vi "Weather_station_main.vi"() -> ()   [LabVIEW 2018]
doc: "通过datasocket技术接收weatherdata发送的数据，之后将数据进行数据显示、数据存储。"
uses:
  variable/weatherdata.vi
  variable/stop.vi
  controls/duoyun.ctl
  controls/dayu.ctl
  controls/sunshine.ctl
panel:
  in  "Array":i8[](array[numeric])
  in  "选项卡控件":enum32{"实时天气显示", "系统结构图"}(tab)
  in  "record":bool caption="停止"
  out "时间":string="21:04"
  in  "地区选择":T1(ring)=enum."金山区"
  out "风速(米/秒)":dbl(knob)=1.2703881999030089 scale=0.0..60.0
  out "风向(度)":dbl(knob)=188.40091984285937 scale=0.0..350.0
  out "气压":dbl(slide)=1004.1359589167787 scale=800.0..1100.0
  out "湿度":dbl(slide)=16.088642176316135 scale=0.0..100.0
  out "温度":dbl(slide)=30.587121929296547 caption="温度(摄氏)" scale=15.0..40.0
  out "雨量(毫米)":dbl(slide)=4.3994523493909 scale=0.0..20.0
  in  "stop":bool caption="停止"
  in  "气象数据更新":bool
  out "日期":string="2007-9-9"
  in  "chongming-sunshine":T2
  in  "chongming-duoyun":T3
  in  "chongming-dayu":T4
  in  "downtown-sunshine":T2
  in  "downtown-dayu":T4
  in  "downtown-duoyun":T3
  in  "jiading-sunshine":T2
  in  "jiading-duoyun":T3
  in  "jiading-dayu":T4
  in  "qinpu-sunshine":T2
  in  "qinpu-duoyun":T3
  in  "qinpu-dayu":T4
  in  "jinshan-sunshine":T2
  in  "jinshan-duoyun":T3
  in  "jiinshan-dayu":T4
  in  "minghang-sunshine":T2
  in  "minghang-duoyun":T3
  in  "minghang-dayu":T4
  in  "pudong-sunshine":T2
  in  "pudong-duoyun":T3
  in  "pudong-dayu":T4
  in  "baoshan-sunshine":T2
  in  "baoshan-duoyun":T3
  in  "baoshan-dayu":T4
  in  "songjiang-sunshine":T2
  in  "songjiang-duoyun":T3
  in  "songjiang-dayu":T4
  in  "fengxian-sunshine":T2
  in  "fengxian-duoyun":T3
  in  "fengxian-dayu":T4
  in  "nanhui-sunshine":T2
  in  "nanhui-hadayu":T4
  in  "nanhui-duoyun":T3
  # "上海地区自动气象站系统"
  # "上海各区实时降雨情况"
  # "上海各区精细天气情况"
  # "气压(百帕)"
  # "相对湿度(%)"
  # "实际——基于cRIO的自动气象站系统"
  # "基于cRIO的自动气象站演示系统是一个分布式的数据采集系统。分布式终端采用NI的cRIO设备对多种气象要素进行采集，并将远程数据通过无线方式送到数据中心计算机进行处理。"
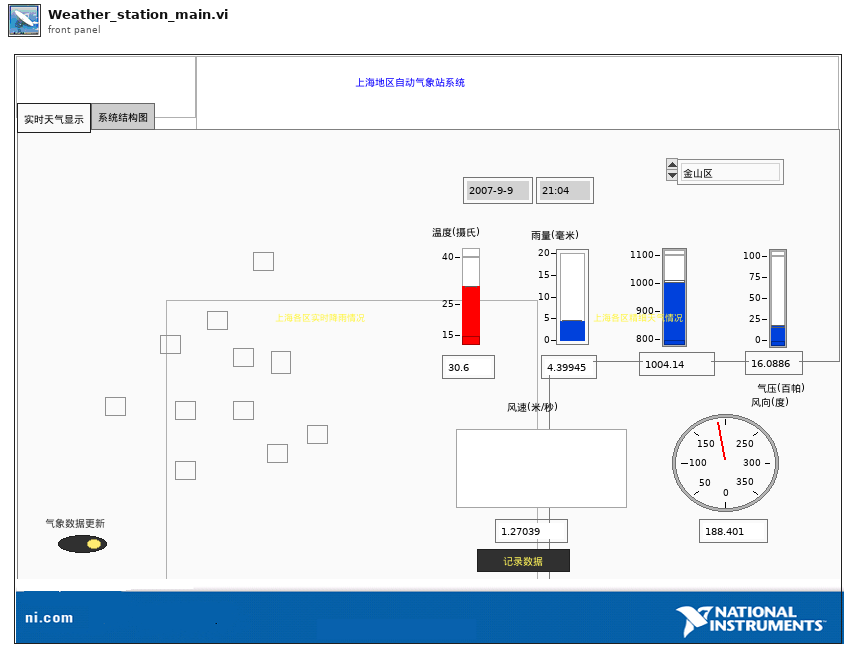
[diagram p1: front panel]
types:
  T1 = enum16{"上海市区", "嘉定区", "青浦区", "金山区", "闵行区", "崇明县", "浦东新区", "宝山区", "松江区", "凤贤区", "南汇区"}
  T2 = typedef "sunshine.ctl" = bool
  T3 = typedef "duoyun.ctl" = bool
  T4 = typedef "dayu.ctl" = bool
  T5 = enum16{"open", "replace", "create", "open or create", "replace or create", "replace or create with confirmation"}
  T6 = cluster{"温度":dbl, "降雨量":dbl, "风向":dbl, "相对湿度":dbl, "气压":dbl, "风速":dbl, "日期":string, "时间":string}[]
  T7 = cluster{"温度":dbl, "降雨量":dbl, "风向":dbl, "相对湿度":dbl, "气压":dbl, "风速":dbl, "日期":string, "时间":string}
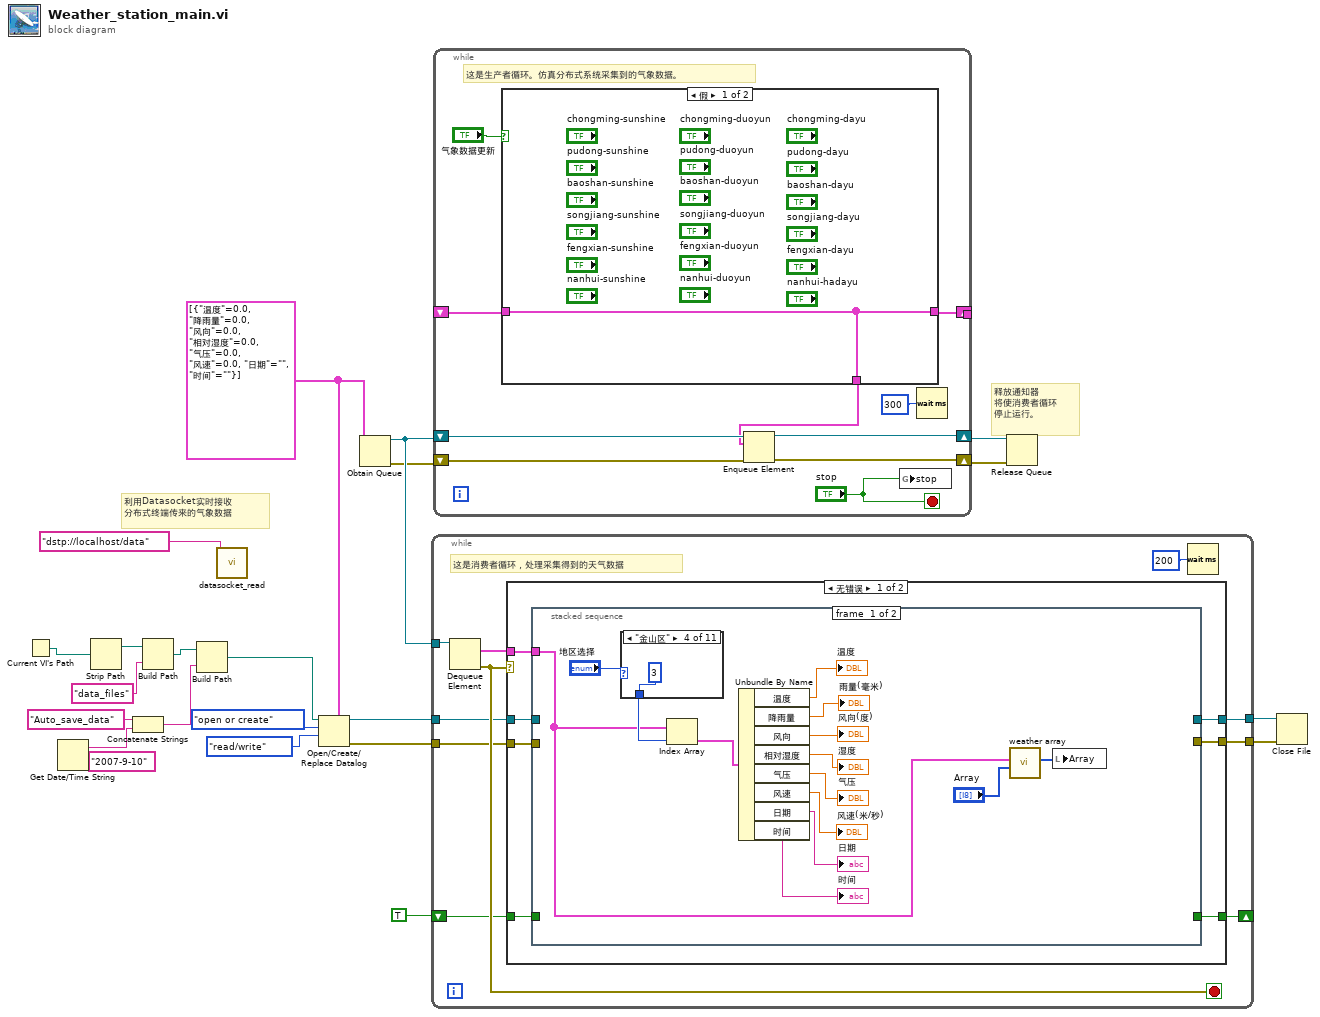
[diagram p0: block diagram]
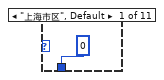
[diagram p2: hidden frame]
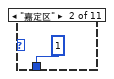
[diagram p3: hidden frame]
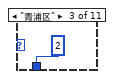
[diagram p4: hidden frame]
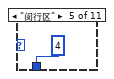
[diagram p5: hidden frame]
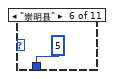
[diagram p6: hidden frame]
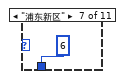
[diagram p7: hidden frame]
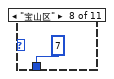
[diagram p8: hidden frame]
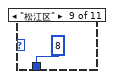
[diagram p9: hidden frame]
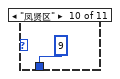
[diagram p10: hidden frame]
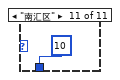
[diagram p11: hidden frame]
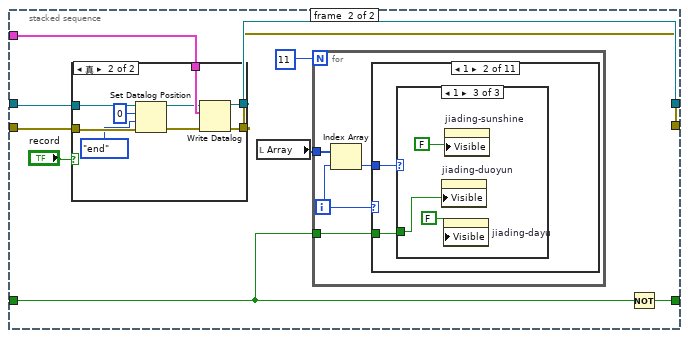
[diagram p12: hidden frame]
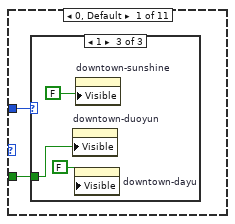
[diagram p13: hidden frame]
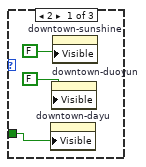
[diagram p14: hidden frame]
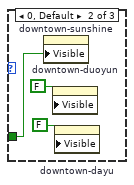
[diagram p15: hidden frame]
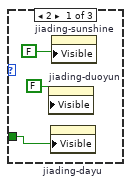
[diagram p16: hidden frame]
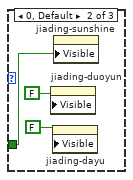
[diagram p17: hidden frame]
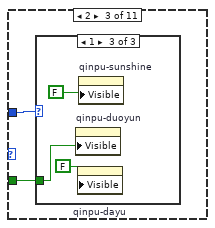
[diagram p18: hidden frame]
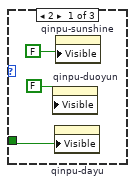
[diagram p19: hidden frame]
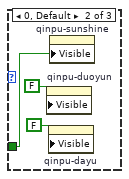
[diagram p20: hidden frame]
diagram:
  (unwired) "2007-9-10" ("字符串")
  w13 = T6 [{"温度"=0.0, "降雨量"=0.0, "风向"=0.0, "相对湿度"=0.0, "气压"=0.0, "风速"=0.0, "日期"="", "时间"=""}]
  # "利用Datasocket实时接收\n分布式终端传来的气象数据"
  # "释放通知器\n将使消费者循环\n停止运行。"
  n1 = Current VI's Path() -> (path=w1:path)
  n2 = Get Date/Time String() -> (date string=w4:string)  [unwired: 3 in, 1 out]
  n3 = Strip Path(path=w1) -> (stripped path=w17:path)  [unwired: 1 out]
  n4 = Concatenate Strings("Auto_save_data" ("字符串"), w4) -> (w5:string)
  n5 = Build Path(base path=w17, name or relative path="data_files" ("名称或相对路径")) -> (appended path=w16:path)
  n6 = Build Path(base path=w16, name or relative path=w5) -> (appended path=w14:path)
  n7 = call "datasocket_read.vi"("URL"="dstp://localhost/data") -> ()  [unwired: 10 in, 1 out]
  n8 = Open/Create/Replace Datalog(5:w13, 9:enum16{"read/write", "read-only", "write-only"}."read/write" ("权限(0:read/write)"), 10:T5."open or create" ("操作(0:open)"), 11:w14) -> (0:w7:errorcluster, 3:w10:refnum<k1>)  [unwired: 2 in, 1 out]
  n9 = Obtain Queue(element data type=w13) -> (queue out=w21:refnum<queue>, error out=w20:errorcluster)  [unwired: 4 in, 1 out]
  n10 = while {
    tunnel: w21 -> [w31]
    tunnel: w10 -> [w28]
    tunnel: w7 -> [w27]
    tunnel: [w26] -> w9
    tunnel: [w25] -> w8
    shift-right: [w24] -> _
    shift-left: TRUE -> [w23]
    stop <- w30 stop-if-true
    # "这是消费者循环，处理采集得到的天气数据"
    n11 = Dequeue Element(queue=w31) -> (element=w29:T6, error out=w30:errorcluster)  [unwired: 2 in, 2 out]
    n12 = case shown="无错误" w30 {
      tunnel: w29 -> [w38 _]
      tunnel: w28 -> [w37 w212]
      tunnel: w27 -> [w36 w211]
      tunnel: [w35 w212] -> w26
      tunnel: [w34 w211] -> w25
      tunnel: [w33 w210] -> w24
      tunnel: w23 -> [w32 w210]
      frame No Error {
        n13 = stacked-sequence {
          tunnel: w38 -> [w41 w71]
          tunnel: w37 -> [_ w70]
          tunnel: w36 -> [_ w69]
          tunnel: [_ w73] -> w35
          tunnel: [_ w72] -> w34
          tunnel: [_ w65] -> w33
          tunnel: w32 -> [_ w64]
          frame #0 {
            n14 = case shown="\"金山区\"" "地区选择" {
              tunnel: [0 1 2 3 4 5 6 7 8 9 10] -> w51
              frame "上海市区", Default {
              }
              frame "嘉定区" {
              }
              frame "青浦区" {
              }
              frame "金山区" {
              }
              frame "闵行区" {
              }
              frame "崇明县" {
              }
              frame "浦东新区" {
              }
              frame "宝山区" {
              }
              frame "松江区" {
              }
              frame "凤贤区" {
              }
              frame "南汇区" {
              }
            }
            n15 = Index Array(array=w41, index=w51) -> (element=w50:T7)
            n16 = Unbundle By Name(w50) -> ("温度"=→"温度":dbl, "降雨量"=→"雨量(毫米)":dbl, "风向"=→"风向(度)":dbl, "相对湿度"=→"湿度":dbl, "气压"=→"气压":dbl, "风速"=→"风速(米/秒)":dbl, "日期"=→"日期":string, "时间"=→"时间":string)
            n17 = call "weather array.vi"("Array"="Array", "数组"=w41) -> ("Array 2"=w39:i8[])  [unwired: 9 in]
            n18 = local write "Array"(w39) -> ()
          }
          frame #1 {
            n19 = case shown="真" "record" {
              tunnel: [w200 w209] -> w73
              tunnel: [w199 w208] -> w72
              tunnel: w71 -> [_ w207]
              tunnel: w70 -> [w200 w206]
              tunnel: w69 -> [w199 w203]
              frame False {
              }
              frame True {
                n20 = Set Datalog Position(4:w203, 5:enum16{"start", "end", "current"}."end" ("自（0：起始）"), 6:i64 0 ("偏移量（记录）（0）"), 7:w206) -> (0:w204:errorcluster, 3:w205:refnum<k1>)
                n21 = Write Datalog(4:w204, 6:w207, 7:w205) -> (0:w208:errorcluster, 3:w209:refnum<k1>)
              }
            }
            n22 = local read "Array"() -> (w67:i8[])
            n23 = for {
              N: 11 -> [_]
              tunnel: w67 -> [w77]
              tunnel: w64 -> [w74]
              i -> [w75]
              n24 = Index Array(array=w77, index=w75) -> (element=w76:i8)
              n25 = case shown="1" w75 {
                tunnel: w76 -> [w79 w90 w101 w112 w123 w134 w145 w156 w167 w178 w189]
                tunnel: w74 -> [w78 w89 w100 w111 w122 w133 w144 w155 w166 w177 w188]
                frame 0, Default {
                  n26 = case shown="1" w79 {
                    tunnel: w78 -> [w80 w83 w86]
                    frame 2 {
                      n27 = property on="downtown-dayu" class="Bool"("Visible"=w80) -> ()  [unwired: 2 in, 2 out]
                      n28 = property on="downtown-duoyun" class="Bool"("Visible"=FALSE) -> ()  [unwired: 2 in, 2 out]
                      n29 = property on="downtown-sunshine" class="Bool"("Visible"=FALSE) -> ()  [unwired: 2 in, 2 out]
                    }
                    frame 0, Default {
                      n30 = property on="downtown-sunshine" class="Bool"("Visible"=w83) -> ()  [unwired: 2 in, 2 out]
                      n31 = property on="downtown-duoyun" class="Bool"("Visible"=FALSE) -> ()  [unwired: 2 in, 2 out]
                      n32 = property on="downtown-dayu" class="Bool"("Visible"=FALSE) -> ()  [unwired: 2 in, 2 out]
                    }
                    frame 1 {
                      n33 = property on="downtown-duoyun" class="Bool"("Visible"=w86) -> ()  [unwired: 2 in, 2 out]
                      n34 = property on="downtown-dayu" class="Bool"("Visible"=FALSE) -> ()  [unwired: 2 in, 2 out]
                      n35 = property on="downtown-sunshine" class="Bool"("Visible"=FALSE) -> ()  [unwired: 2 in, 2 out]
                    }
                  }
                }
                frame 1 {
                  n36 = case shown="1" w90 {
                    tunnel: w89 -> [w91 w94 w97]
                    frame 2 {
                      n37 = property on="jiading-duoyun" class="Bool"("Visible"=FALSE) -> ()  [unwired: 2 in, 2 out]
                      n38 = property on="jiading-dayu" class="Bool"("Visible"=w91) -> ()  [unwired: 2 in, 2 out]
                      n39 = property on="jiading-sunshine" class="Bool"("Visible"=FALSE) -> ()  [unwired: 2 in, 2 out]
                    }
                    frame 0, Default {
                      n40 = property on="jiading-duoyun" class="Bool"("Visible"=FALSE) -> ()  [unwired: 2 in, 2 out]
                      n41 = property on="jiading-dayu" class="Bool"("Visible"=FALSE) -> ()  [unwired: 2 in, 2 out]
                      n42 = property on="jiading-sunshine" class="Bool"("Visible"=w94) -> ()  [unwired: 2 in, 2 out]
                    }
                    frame 1 {
                      n43 = property on="jiading-duoyun" class="Bool"("Visible"=w97) -> ()  [unwired: 2 in, 2 out]
                      n44 = property on="jiading-dayu" class="Bool"("Visible"=FALSE) -> ()  [unwired: 2 in, 2 out]
                      n45 = property on="jiading-sunshine" class="Bool"("Visible"=FALSE) -> ()  [unwired: 2 in, 2 out]
                    }
                  }
                }
                frame 2 {
                  n46 = case shown="1" w101 {
                    tunnel: w100 -> [w102 w105 w108]
                    frame 2 {
                      n47 = property on="qinpu-duoyun" class="Bool"("Visible"=FALSE) -> ()  [unwired: 2 in, 2 out]
                      n48 = property on="qinpu-dayu" class="Bool"("Visible"=w102) -> ()  [unwired: 2 in, 2 out]
                      n49 = property on="qinpu-sunshine" class="Bool"("Visible"=FALSE) -> ()  [unwired: 2 in, 2 out]
                    }
                    frame 0, Default {
                      n50 = property on="qinpu-duoyun" class="Bool"("Visible"=FALSE) -> ()  [unwired: 2 in, 2 out]
                      n51 = property on="qinpu-dayu" class="Bool"("Visible"=FALSE) -> ()  [unwired: 2 in, 2 out]
                      n52 = property on="qinpu-sunshine" class="Bool"("Visible"=w105) -> ()  [unwired: 2 in, 2 out]
                    }
                    frame 1 {
                      n53 = property on="qinpu-duoyun" class="Bool"("Visible"=w108) -> ()  [unwired: 2 in, 2 out]
                      n54 = property on="qinpu-dayu" class="Bool"("Visible"=FALSE) -> ()  [unwired: 2 in, 2 out]
                      n55 = property on="qinpu-sunshine" class="Bool"("Visible"=FALSE) -> ()  [unwired: 2 in, 2 out]
                    }
                  }
                }
                frame 3 {
                  n56 = case shown="2" w112 {
                    tunnel: w111 -> [w113 w116 w119]
                    frame 2 {
                      n57 = property on="jinshan-duoyun" class="Bool"("Visible"=FALSE) -> ()  [unwired: 2 in, 2 out]
                      n58 = property on="jiinshan-dayu" class="Bool"("Visible"=w113) -> ()  [unwired: 2 in, 2 out]
                      n59 = property on="jinshan-sunshine" class="Bool"("Visible"=FALSE) -> ()  [unwired: 2 in, 2 out]
                    }
                    frame 0, Default {
                      n60 = property on="jinshan-duoyun" class="Bool"("Visible"=FALSE) -> ()  [unwired: 2 in, 2 out]
                      n61 = property on="jiinshan-dayu" class="Bool"("Visible"=FALSE) -> ()  [unwired: 2 in, 2 out]
                      n62 = property on="jinshan-sunshine" class="Bool"("Visible"=w116) -> ()  [unwired: 2 in, 2 out]
                    }
                    frame 1 {
                      n63 = property on="jinshan-duoyun" class="Bool"("Visible"=w119) -> ()  [unwired: 2 in, 2 out]
                      n64 = property on="jiinshan-dayu" class="Bool"("Visible"=FALSE) -> ()  [unwired: 2 in, 2 out]
                      n65 = property on="jinshan-sunshine" class="Bool"("Visible"=FALSE) -> ()  [unwired: 2 in, 2 out]
                    }
                  }
                }
                frame 4 {
                  n66 = case shown="2" w123 {
                    tunnel: w122 -> [w124 w127 w130]
                    frame 2 {
                      n67 = property on="minghang-duoyun" class="Bool"("Visible"=FALSE) -> ()  [unwired: 2 in, 2 out]
                      n68 = property on="minghang-dayu" class="Bool"("Visible"=w124) -> ()  [unwired: 2 in, 2 out]
                      n69 = property on="minghang-sunshine" class="Bool"("Visible"=FALSE) -> ()  [unwired: 2 in, 2 out]
                    }
                    frame 0, Default {
                      n70 = property on="minghang-duoyun" class="Bool"("Visible"=FALSE) -> ()  [unwired: 2 in, 2 out]
                      n71 = property on="minghang-dayu" class="Bool"("Visible"=FALSE) -> ()  [unwired: 2 in, 2 out]
                      n72 = property on="minghang-sunshine" class="Bool"("Visible"=w127) -> ()  [unwired: 2 in, 2 out]
                    }
                    frame 1 {
                      n73 = property on="minghang-duoyun" class="Bool"("Visible"=w130) -> ()  [unwired: 2 in, 2 out]
                      n74 = property on="minghang-dayu" class="Bool"("Visible"=FALSE) -> ()  [unwired: 2 in, 2 out]
                      n75 = property on="minghang-sunshine" class="Bool"("Visible"=FALSE) -> ()  [unwired: 2 in, 2 out]
                    }
                  }
                }
                frame 5 {
                  n76 = case shown="1" w134 {
                    tunnel: w133 -> [w135 w138 w142]
                    frame 2 {
                      n77 = property on="chongming-duoyun" class="Bool"("Visible"=FALSE) -> ()  [unwired: 2 in, 2 out]
                      n78 = property on="chongming-dayu" class="Bool"("Visible"=w135) -> ()  [unwired: 2 in, 2 out]
                      n79 = property on="chongming-sunshine" class="Bool"("Visible"=FALSE) -> ()  [unwired: 2 in, 2 out]
                    }
                    frame 0, Default {
                      n80 = property on="chongming-sunshine" class="Bool"("Visible"=w138) -> ()  [unwired: 2 in, 2 out]
                      n81 = property on="chongming-duoyun" class="Bool"("Visible"=FALSE) -> ()  [unwired: 2 in, 2 out]
                      n82 = property on="chongming-dayu" class="Bool"("Visible"=FALSE) -> ()  [unwired: 2 in, 2 out]
                    }
                    frame 1 {
                      n83 = property on="chongming-sunshine" class="Bool"("Visible"=FALSE) -> ()  [unwired: 2 in, 2 out]
                      n84 = property on="chongming-duoyun" class="Bool"("Visible"=w142) -> ()  [unwired: 2 in, 2 out]
                      n85 = property on="chongming-dayu" class="Bool"("Visible"=FALSE) -> ()  [unwired: 2 in, 2 out]
                    }
                  }
                }
                frame 7 {
                  n86 = case shown="1" w145 {
                    tunnel: w144 -> [w146 w149 w152]
                    frame 2 {
                      n87 = property on="baoshan-duoyun" class="Bool"("Visible"=FALSE) -> ()  [unwired: 2 in, 2 out]
                      n88 = property on="baoshan-dayu" class="Bool"("Visible"=w146) -> ()  [unwired: 2 in, 2 out]
                      n89 = property on="baoshan-sunshine" class="Bool"("Visible"=FALSE) -> ()  [unwired: 2 in, 2 out]
                    }
                    frame 0, Default {
                      n90 = property on="baoshan-duoyun" class="Bool"("Visible"=FALSE) -> ()  [unwired: 2 in, 2 out]
                      n91 = property on="baoshan-dayu" class="Bool"("Visible"=FALSE) -> ()  [unwired: 2 in, 2 out]
                      n92 = property on="baoshan-sunshine" class="Bool"("Visible"=w149) -> ()  [unwired: 2 in, 2 out]
                    }
                    frame 1 {
                      n93 = property on="baoshan-duoyun" class="Bool"("Visible"=w152) -> ()  [unwired: 2 in, 2 out]
                      n94 = property on="baoshan-dayu" class="Bool"("Visible"=FALSE) -> ()  [unwired: 2 in, 2 out]
                      n95 = property on="baoshan-sunshine" class="Bool"("Visible"=FALSE) -> ()  [unwired: 2 in, 2 out]
                    }
                  }
                }
                frame 8 {
                  n96 = case shown="1" w156 {
                    tunnel: w155 -> [w157 w160 w163]
                    frame 2 {
                      n97 = property on="songjiang-duoyun" class="Bool"("Visible"=FALSE) -> ()  [unwired: 2 in, 2 out]
                      n98 = property on="songjiang-dayu" class="Bool"("Visible"=w157) -> ()  [unwired: 2 in, 2 out]
                      n99 = property on="songjiang-sunshine" class="Bool"("Visible"=FALSE) -> ()  [unwired: 2 in, 2 out]
                    }
                    frame 0, Default {
                      n100 = property on="songjiang-duoyun" class="Bool"("Visible"=FALSE) -> ()  [unwired: 2 in, 2 out]
                      n101 = property on="songjiang-dayu" class="Bool"("Visible"=FALSE) -> ()  [unwired: 2 in, 2 out]
                      n102 = property on="songjiang-sunshine" class="Bool"("Visible"=w160) -> ()  [unwired: 2 in, 2 out]
                    }
                    frame 1 {
                      n103 = property on="songjiang-duoyun" class="Bool"("Visible"=w163) -> ()  [unwired: 2 in, 2 out]
                      n104 = property on="songjiang-dayu" class="Bool"("Visible"=FALSE) -> ()  [unwired: 2 in, 2 out]
                      n105 = property on="songjiang-sunshine" class="Bool"("Visible"=FALSE) -> ()  [unwired: 2 in, 2 out]
                    }
                  }
                }
                frame 9 {
                  n106 = case shown="2" w167 {
                    tunnel: w166 -> [w168 w171 w174]
                    frame 2 {
                      n107 = property on="fengxian-duoyun" class="Bool"("Visible"=FALSE) -> ()  [unwired: 2 in, 2 out]
                      n108 = property on="fengxian-dayu" class="Bool"("Visible"=w168) -> ()  [unwired: 2 in, 2 out]
                      n109 = property on="fengxian-sunshine" class="Bool"("Visible"=FALSE) -> ()  [unwired: 2 in, 2 out]
                    }
                    frame 0, Default {
                      n110 = property on="fengxian-duoyun" class="Bool"("Visible"=FALSE) -> ()  [unwired: 2 in, 2 out]
                      n111 = property on="fengxian-dayu" class="Bool"("Visible"=FALSE) -> ()  [unwired: 2 in, 2 out]
                      n112 = property on="fengxian-sunshine" class="Bool"("Visible"=w171) -> ()  [unwired: 2 in, 2 out]
                    }
                    frame 1 {
                      n113 = property on="fengxian-duoyun" class="Bool"("Visible"=w174) -> ()  [unwired: 2 in, 2 out]
                      n114 = property on="fengxian-dayu" class="Bool"("Visible"=FALSE) -> ()  [unwired: 2 in, 2 out]
                      n115 = property on="fengxian-sunshine" class="Bool"("Visible"=FALSE) -> ()  [unwired: 2 in, 2 out]
                    }
                  }
                }
                frame 10 {
                  n116 = case shown="0, 默认" w178 {
                    tunnel: w177 -> [w179 w182 w185]
                    frame 2 {
                      n117 = property on="nanhui-duoyun" class="Bool"("Visible"=FALSE) -> ()  [unwired: 2 in, 2 out]
                      n118 = property on="nanhui-hadayu" class="Bool"("Visible"=w179) -> ()  [unwired: 2 in, 2 out]
                      n119 = property on="nanhui-sunshine" class="Bool"("Visible"=FALSE) -> ()  [unwired: 2 in, 2 out]
                    }
                    frame 0, Default {
                      n120 = property on="nanhui-duoyun" class="Bool"("Visible"=FALSE) -> ()  [unwired: 2 in, 2 out]
                      n121 = property on="nanhui-hadayu" class="Bool"("Visible"=FALSE) -> ()  [unwired: 2 in, 2 out]
                      n122 = property on="nanhui-sunshine" class="Bool"("Visible"=w182) -> ()  [unwired: 2 in, 2 out]
                    }
                    frame 1 {
                      n123 = property on="nanhui-duoyun" class="Bool"("Visible"=w185) -> ()  [unwired: 2 in, 2 out]
                      n124 = property on="nanhui-hadayu" class="Bool"("Visible"=FALSE) -> ()  [unwired: 2 in, 2 out]
                      n125 = property on="nanhui-sunshine" class="Bool"("Visible"=FALSE) -> ()  [unwired: 2 in, 2 out]
                    }
                  }
                }
                frame 6 {
                  n126 = case shown="1" w189 {
                    tunnel: w188 -> [w190 w193 w196]
                    frame 2 {
                      n127 = property on="pudong-duoyun" class="Bool"("Visible"=FALSE) -> ()  [unwired: 2 in, 2 out]
                      n128 = property on="pudong-dayu" class="Bool"("Visible"=w190) -> ()  [unwired: 2 in, 2 out]
                      n129 = property on="pudong-sunshine" class="Bool"("Visible"=FALSE) -> ()  [unwired: 2 in, 2 out]
                    }
                    frame 0, Default {
                      n130 = property on="pudong-duoyun" class="Bool"("Visible"=FALSE) -> ()  [unwired: 2 in, 2 out]
                      n131 = property on="pudong-dayu" class="Bool"("Visible"=FALSE) -> ()  [unwired: 2 in, 2 out]
                      n132 = property on="pudong-sunshine" class="Bool"("Visible"=w193) -> ()  [unwired: 2 in, 2 out]
                    }
                    frame 1 {
                      n133 = property on="pudong-duoyun" class="Bool"("Visible"=w196) -> ()  [unwired: 2 in, 2 out]
                      n134 = property on="pudong-dayu" class="Bool"("Visible"=FALSE) -> ()  [unwired: 2 in, 2 out]
                      n135 = property on="pudong-sunshine" class="Bool"("Visible"=FALSE) -> ()  [unwired: 2 in, 2 out]
                    }
                  }
                }
              }
            }
            n136 = Not(x=w64) -> (.not. x?=w65:bool)
          }
        }
      }
      frame Error {
      }
    }
    n137 = Wait (ms)(milliseconds to wait=u32 200) -> ()  [unwired: 1 out]
  }
  n138 = while {
    shift-right: [w219] -> w18
    shift-left: w20 -> [w220]
    shift-right: [w221] -> w19
    shift-left: w21 -> [w222]
    tunnel: [w215] -> _
    shift-right: [w215] -> _
    shift-left: _ -> [w214]
    stop <- "stop" stop-if-true
    # "这是生产者循环。仿真分布式系统采集到的气象数据。"
    n139 = case shown="假" "气象数据更新" {
      tunnel: [w223 w224] -> w216
      tunnel: [w223 w224] -> w215
      tunnel: w214 -> [w223 _]
      frame False {
      }
      frame True {
        n140 = global read "weatherdata.vi" "数据"() -> (w224:T6)
      }
    }
    n141 = Enqueue Element(queue=w222, element=w216, error in (no error)=w220) -> (queue out=w221:refnum<queue>, error out=w219:errorcluster)  [unwired: 1 in, 1 out]
    n142 = global write "stop.vi" "stop"("stop") -> ()
    n143 = Wait (ms)(milliseconds to wait=u32 300) -> ()  [unwired: 1 out]
  }
  n144 = Release Queue(queue=w19, error in (no error)=w18) -> ()  [unwired: 1 in, 3 out]
  n145 = Close File(refnum=w9, error in=w8) -> ()  [unwired: 2 out]
